vi "Colorcycle2002.vi"   [LabVIEW 2013]
uses:
  <vilib>/Heliosphere Research LLC/Advanced Plotting Toolkit/api_annotations/LegendPositions.ctl
  <vilib>/Heliosphere Research LLC/Advanced Plotting Toolkit/Advanced Plotting Toolkit.lvlib
types:
  T1 = typedef "Advanced Plotting Toolkit.lvlib/LegendPositions.ctl" = enum16{"Default", "Top Right", "Top", "Top Left", "Left", "Bottom Left", "Bottom", "Bottom Right", "Right", "Center"}
  T2 = typedef "Advanced Plotting Toolkit.lvlib/PlotID.ctl" = i32
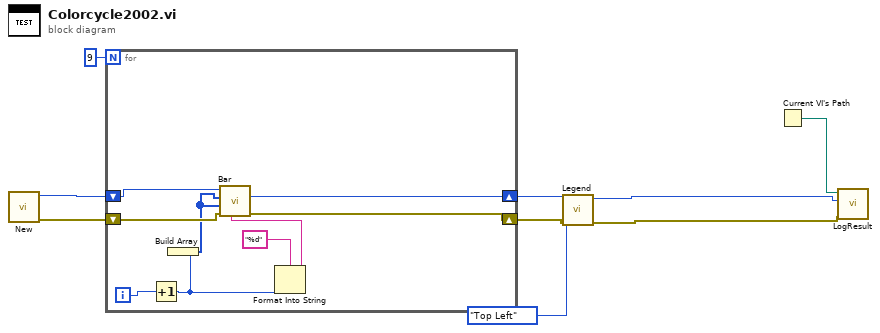
[diagram p0: block diagram]
diagram:
  n1 = call <vilib>:"New.vi"() -> ("error out"=w7:errorcluster, "Plot ID"=w8:T2)  [unwired: 10 in]
  n2 = for {
    N: 9 -> [_]
    shift-right: [w15] -> w6
    shift-left: w8 -> [w18]
    shift-right: [w16] -> w4
    shift-left: w7 -> [w17]
    i -> [w14]
    n3 = Increment(x=w14) -> (x+1=w11:i32)
    n4 = Build Array(w11) -> (w10:i32[])
    n5 = Format Into String(format string="%d", w11) -> (resulting string=w12:string)  [unwired: 2 in, 1 out]
    n6 = call <vilib>:"Bar.vi"("Legend Title"=w12, "error in (no error)"=w17, "Bar Lengths"=w10, "X Coordinates"=w10, "Plot ID"=w18) -> ("error out"=w16:errorcluster, "Plot ID Out"=w15:T2)  [unwired: 5 in]
  }
  n7 = call <vilib>:"Legend.vi"("error in (no error)"=w4, "Position"=LegendPositions."Top Left", "Plot ID"=w6) -> ("error out"=w3:errorcluster, "Plot ID Out"=w5:T2)  [unwired: 7 in]
  n8 = Current VI's Path() -> (path=w9:path)
  n9 = call "LogResult.vi"("Test Result"=w3, "Test Artifact"=w5, "VI Path"=w9) -> ()  [unwired: 9 in]
